vi "主程序.vi"() -> ()   [LabVIEW 2012]
panel:
  in  "数组":cluster{"x":dbl, "y":dbl}[](array[cluster])
  in  "图片":picture
  in  "状态":bool=TRUE
  in  "食物位置":cluster{"x":dbl, "y":dbl}
  in  "行列数":i32
  in  "点":cluster{"x":dbl, "y":dbl}
  in  "网格大小":dbl
  out "食物":bool
  in  "方向":i32
  out "new picture":picture
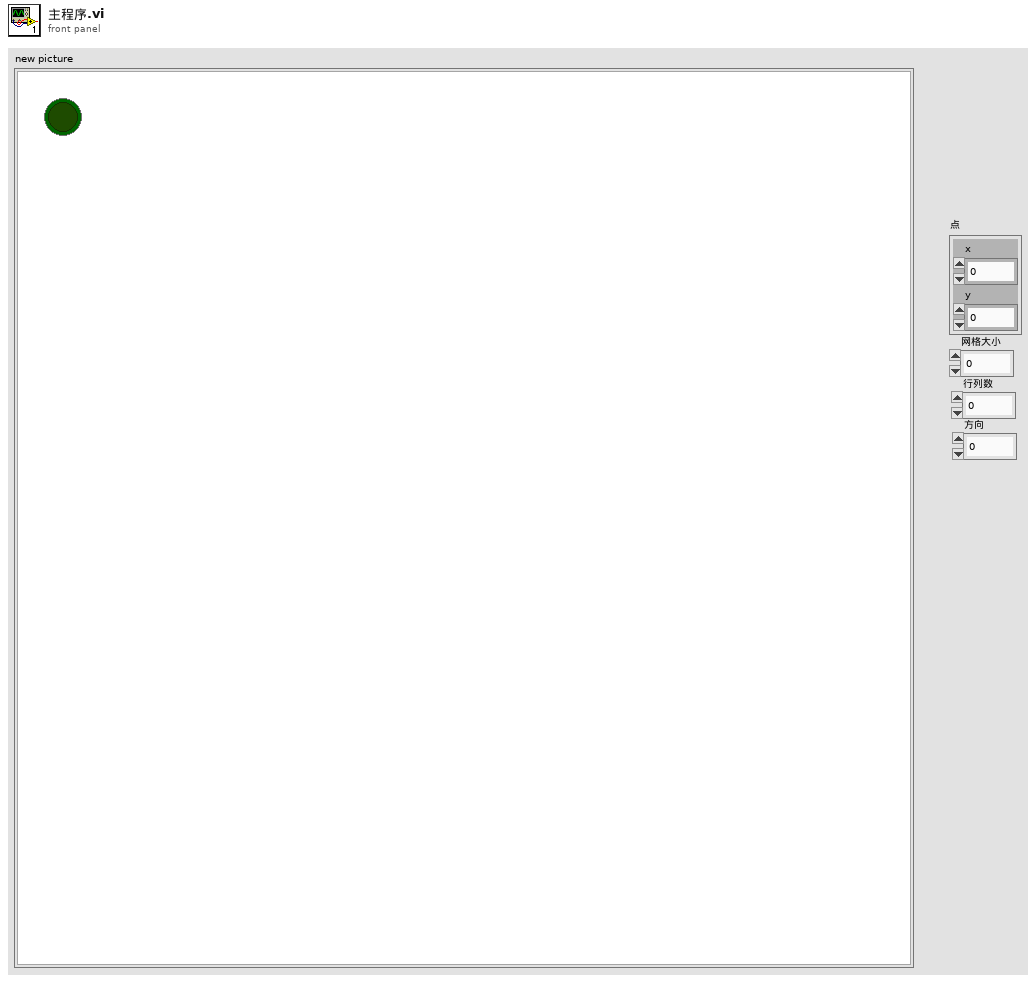
[diagram p1: front panel]
types:
  T1 = typedef "eventvkey.ctl" = enum16{"ASCII", "Enter", "Return", "Shift", "Ctrl", "Alt", "Cmd", "Opt", "Caps", "NumLock", "Clear", "Break", "Up", "Down", "Left", "Right", "Insert", "Delete", "Home", "End", "PageUp", "PageDown", "Escape", "Help", "Pause", "ScrollLock", "F1", "F2", "F3", "F4", "F5", "F6", "F7", "F8", "F9", "F10", "F11", "F12", "F13", "F14", "F15", "F16", "F17", "F18", "F19", "F20", "F21", "F22", "F23", "F24", "Play", "VolumeUp", "VolumeDown", "Mute", "Two Byte Char"}
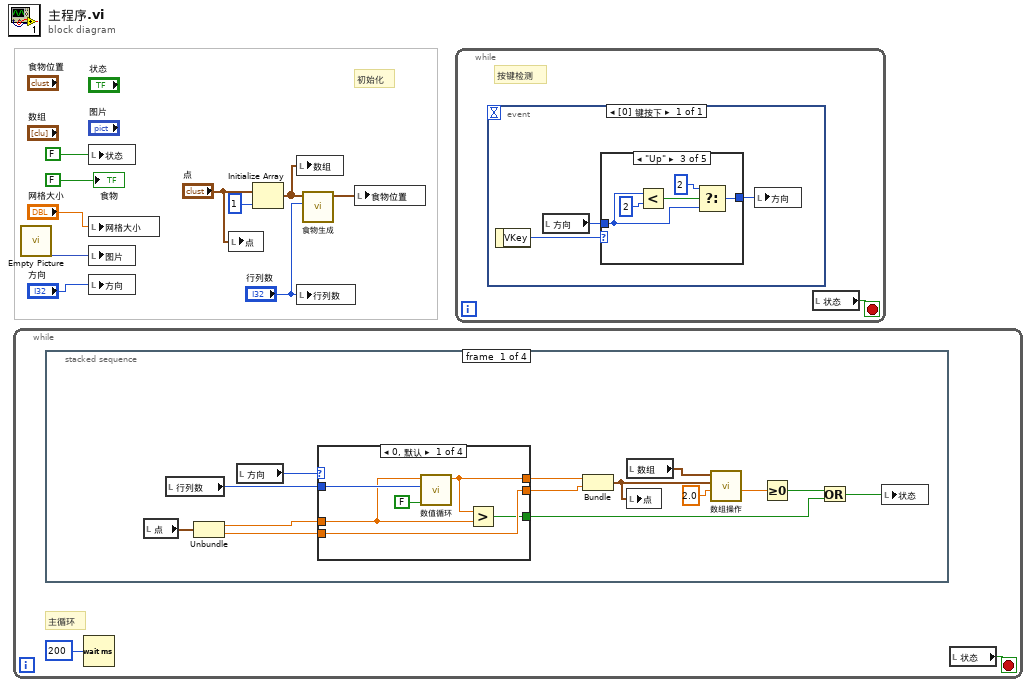
[diagram p0: block diagram]
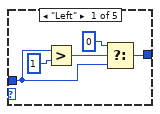
[diagram p2: hidden frame]
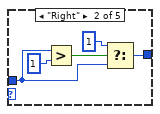
[diagram p3: hidden frame]
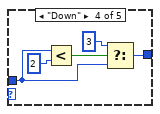
[diagram p4: hidden frame]
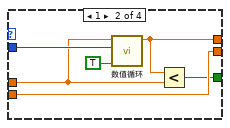
[diagram p6: hidden frame]
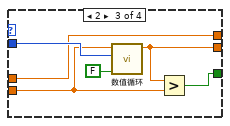
[diagram p7: hidden frame]
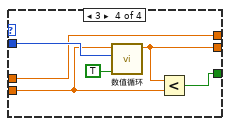
[diagram p8: hidden frame]
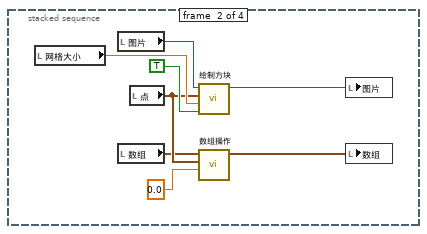
[diagram p9: hidden frame]
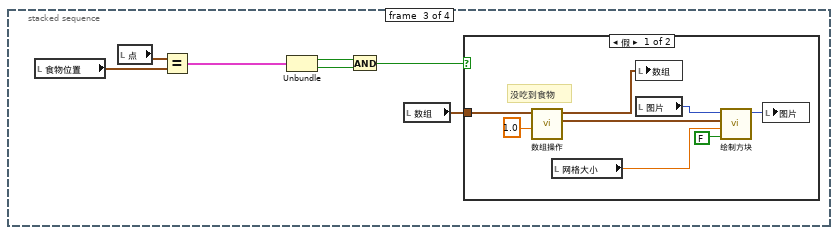
[diagram p10: hidden frame]
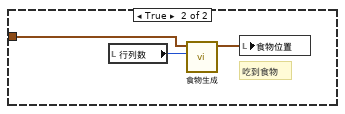
[diagram p11: hidden frame]
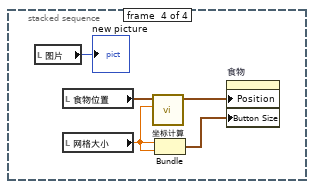
[diagram p12: hidden frame]
diagram:
  # "初始化"
  n1 = while {
    stop <- w11 stop-if-true
    # "主循环"
    n2 = stacked-sequence {
      frame #0 {
        n3 = local read "点"() -> (w26:cluster{"x":dbl, "y":dbl})
        n4 = local read "行列数"() -> (w22:i32)
        n5 = Unbundle(w26) -> ("x"=w24:dbl, "y"=w23:dbl)
        n6 = local read "方向"() -> (w21:i32)
        n7 = case shown="0, 默认" w21 {
          tunnel: w24 -> [w29 w34 w42 w48]
          tunnel: w23 -> [w30 w37 w40 w46]
          tunnel: [w28 w35 w42 w48] -> w20
          tunnel: [w30 w37 w39 w45] -> w19
          tunnel: w22 -> [w31 w36 w43 w49]
          tunnel: [w27 w33 w41 w47] -> w15
          frame 0, Default {
            n8 = call "数值循环.vi"("加/减"=FALSE, "上限"=w31, "输入"=w29) -> ("输出"=w28:dbl)  [unwired: 8 in]
            n9 = Greater?(x=w28, y=w29) -> (0:w27:bool)
          }
          frame 1 {
            n10 = call "数值循环.vi"("加/减"=TRUE, "上限"=w36, "输入"=w34) -> ("输出"=w35:dbl)  [unwired: 8 in]
            n11 = Less?(x=w35, y=w34) -> (x < y?=w33:bool)
          }
          frame 2 {
            n12 = call "数值循环.vi"("加/减"=FALSE, "上限"=w43, "输入"=w40) -> ("输出"=w39:dbl)  [unwired: 8 in]
            n13 = Greater?(x=w39, y=w40) -> (0:w41:bool)
          }
          frame 3 {
            n14 = call "数值循环.vi"("加/减"=TRUE, "上限"=w49, "输入"=w46) -> ("输出"=w45:dbl)  [unwired: 8 in]
            n15 = Less?(x=w45, y=w46) -> (x < y?=w47:bool)
          }
        }
        n16 = Bundle("x"=w20, "输出"=w19) -> (w25:cluster{"x":dbl, "输出":dbl})  [unwired: 1 in]
        n17 = local read "数组"() -> (w18:cluster{"x":dbl, "y":dbl}[])
        n18 = local write "点"(w25) -> ()
        n19 = call "数组操作.vi"("操作码"=2.0, "输入点"=w25, "数组输入"=w18) -> ("索引"=w16:dbl)  [unwired: 6 in, 2 out]
        n20 = Greater Or Equal To 0?(x=w16) -> (x >= 0?=w14:bool)
        n21 = Or(x=w14, y=w15) -> (x .or. y?=w13:bool)
        n22 = local write "状态"(w13) -> ()
      }
      frame #1 {
        n23 = local read "网格大小"() -> (w56:dbl)
        n24 = local read "图片"() -> (w55:picture)
        n25 = local read "数组"() -> (w52:cluster{"x":dbl, "y":dbl}[])
        n26 = local read "点"() -> (w53:cluster{"x":dbl, "y":dbl})
        n27 = call "绘制方块.vi"("绘制/清除"=TRUE, "网格大小"=w56, "输入点"=w53, "picture"=w55) -> ("new picture"=w54:picture)  [unwired: 7 in]
        n28 = call "数组操作.vi"("操作码"=0.0, "输入点"=w53, "数组输入"=w52) -> ("数组输出"=w51:cluster{"x":dbl, "y":dbl}[])  [unwired: 6 in, 2 out]
        n29 = local write "图片"(w54) -> ()
        n30 = local write "数组"(w51) -> ()
      }
      frame #2 {
        n31 = local read "食物位置"() -> (w65:cluster{"x":dbl, "y":dbl})
        n32 = local read "点"() -> (w63:cluster{"x":dbl, "y":dbl})
        n33 = Equal?(x=w63, y=w65) -> (x = y?=w64:cluster{"x":bool, "y":bool})
        n34 = Unbundle(w64) -> ("x"=w60:bool, "y"=w61:bool)
        n35 = And(x=w60, y=w61) -> (x .and. y?=w59:bool)
        n36 = local read "数组"() -> (w62:cluster{"x":dbl, "y":dbl}[])
        n37 = case shown="假" w59 {
          tunnel: w62 -> [w70 w74]
          frame False {
            # "没吃到食物"
            n38 = call "数组操作.vi"("操作码"=1.0, "数组输入"=w70) -> ("输出点"=w72:cluster{"x":dbl, "y":dbl}, "数组输出"=w67:cluster{"x":dbl, "y":dbl}[])  [unwired: 7 in, 1 out]
            n39 = local read "网格大小"() -> (w66:dbl)
            n40 = local write "数组"(w67) -> ()
            n41 = local read "图片"() -> (w69:picture)
            n42 = call "绘制方块.vi"("绘制/清除"=FALSE, "网格大小"=w66, "输入点"=w72, "picture"=w69) -> ("new picture"=w68:picture)  [unwired: 7 in]
            n43 = local write "图片"(w68) -> ()
          }
          frame True {
            # "吃到食物"
            n44 = local read "行列数"() -> (w75:i32)
            n45 = call "食物生成.vi"("上限"=w75, "数组输入"=w74) -> ("输出点"=w76:cluster{"x":dbl, "y":dbl})  [unwired: 9 in]
            n46 = local write "食物位置"(w76) -> ()
          }
        }
      }
      frame #3 {
        n47 = local read "图片"() -> (→"new picture":picture)
        n48 = local read "食物位置"() -> (w79:cluster{"x":dbl, "y":dbl})
        n49 = local read "网格大小"() -> (w80:dbl)
        n50 = call "坐标计算.vi"("网格大小"=w80, "输入"=w79) -> ("输出"=w78:cluster{"x":dbl, "y":dbl})  [unwired: 9 in]
        n51 = Bundle("网格大小"=w80, "网格大小"=w80) -> (w81:cluster{"网格大小":dbl, "网格大小":dbl})  [unwired: 1 in]
        n52 = property on="食物" class="Bool (严格)"("Position"=w78, "Button Size"=w81) -> ()  [unwired: 2 in, 2 out]
      }
    }
    n53 = Wait (ms)(milliseconds to wait=u32 200 ("等待时间（毫秒）")) -> ()  [unwired: 1 out]
    n54 = local read "状态"() -> (w11:bool)
  }
  n55 = call "Empty Picture"() -> ("empty picture"=w4:picture)
  n56 = local write "状态"(FALSE ("状态")) -> ()
  n57 = local write "网格大小"("网格大小") -> ()
  n58 = local write "图片"(w4) -> ()
  n59 = local write "方向"("方向") -> ()
  n60 = local write "点"("点") -> ()
  n61 = Initialize Array("点", 1 ("维数大小")) -> (w6:cluster{"x":dbl, "y":dbl}[])
  n62 = local write "数组"(w6) -> ()
  n63 = local write "行列数"("行列数") -> ()
  n64 = call "食物生成.vi"("上限"="行列数", "数组输入"=w6) -> ("输出点"=w8:cluster{"x":dbl, "y":dbl})  [unwired: 9 in]
  n65 = local write "食物位置"(w8) -> ()
  n66 = while {
    stop <- w82 stop-if-true
    # "按键检测"
    n67 = event shown="[0] 键按下" {
      selector: _ -> [_]
      dyn-events: _ -> [_]
      timeout: _ -> [_]
      event Key Down {
        n68 = event-data() -> ("VKey"=w85:T1)  [unwired: 1 in]
        n69 = local read "方向"() -> (w84:i32)
        n70 = case shown="\"Up\"" w85 {
          tunnel: w84 -> [w87 w92 w97 w102 w106]
          tunnel: [w86 w91 w96 w101 w106] -> w83
          frame "Left" {
            n71 = Greater?(x=w87, y=1) -> (0:w89:bool)
            n72 = Select(t=u16 0, s=w89, f=w87) -> (s? t:f=w86:i32)
          }
          frame "Right" {
            n73 = Greater?(x=w92, y=1) -> (0:w94:bool)
            n74 = Select(t=u16 1, s=w94, f=w92) -> (s? t:f=w91:i32)
          }
          frame "Up" {
            n75 = Less?(x=w97, y=2) -> (x < y?=w99:bool)
            n76 = Select(t=u16 2, s=w99, f=w97) -> (s? t:f=w96:i32)
          }
          frame "Down" {
            n77 = Less?(x=w102, y=2) -> (x < y?=w104:bool)
            n78 = Select(t=u16 3, s=w104, f=w102) -> (s? t:f=w101:i32)
          }
          frame "ASCII", Default {
          }
        }
        n79 = local write "方向"(w83) -> ()
      }
    }
    n80 = local read "状态"() -> (w82:bool)
  }
  "食物" <- FALSE ("食物")
